vi "INIT swerve.vi"(8 "error in (no error)":errorcluster) -> (0 "error out":errorcluster)   [LabVIEW 2023]
uses:
  <vilib>/Rock Robotics/WPI/ThirdParty/REV Robotics/REVLib/Typedef/Spark MAX Control Type.ctl
  Global INIT.vi
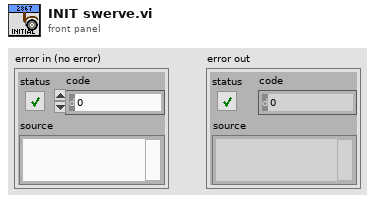
[diagram p1: front panel]
types:
  T1 = typedef "ctrl swerve motor.ctl" = cluster{"description":string, "MOTOR SELECT":T2, "Installed?":bool, "CAN ID":u8, "refnum name":string, "Invert":bool, "Idle Mode":T3, "Current limiting":T4, "MOTOR PIDF coefficients":T5, "gear ratio":dbl}
  T2 = typedef "ctrl MOTOR SELECT.ctl" = i16
  T3 = typedef "Spark MAX Idle Mode.ctl" = enum16{"Coast", "Brake"}
  T4 = typedef "ctrl Spark MAX current limiting.ctl" = cluster{"Linearized":bool, "Free Speed (A)":dbl, "Primay (A)":dbl, "Limit RPM (0)":u32}
  T5 = typedef "ctrl motor PIDF coefficients.ctl" = cluster{"PIDF":cluster{"P Gain":dbl, "I Gain":dbl, "D Gain":dbl, "F Gain":dbl, "I Zone":dbl, "Min Output":dbl, "Max Output":dbl}, "Smart Motion":T6}
  T6 = typedef "Spark MAX Smart Motion Parameters.ctl" = cluster{"Max Velocity":dbl, "Max Acceleration":dbl, "Minimum Velocity Output":dbl, "Allowed Closed Loop Error":dbl}
  T7 = typedef "ctrl CANcoder.ctl" = cluster{"description":string, "Installed?":bool, "CAN ID":u8, "CAN Bus":string, "refnum name":string, "Sensor Direction":bool, "Magnet Offset (Degrees)":dbl, "gear ratio":dbl}
  T8 = typedef "Spark MAX Control Type.ctl" = enum16{"Percent VBus", "Voltage", "Velocity", "Position", "Smart Motion", "Current", "Smart Velocity"}
  T9 = typedef "WPI_MotorControlDeviceRef.ctl" = cluster{"DeviceStatus":errorcluster, "Type":T10, "PWM":cluster{"PWM Channel":T11, "DeadBand":T12}, "CAN":cluster{"Device Number":u8, "SetOutput VI Ref":variant, "GetOutput VI Ref":variant, "Enable VI Ref":variant, "Disable VI Ref":variant, "Data":variant}, "Invert":bool, "DIO PWM":cluster{"PWM \"Enable\" Channel":T11, "DIOChannel":T13, "PWM Rate":dbl}}
  T10 = typedef "WPI_MotorControlType.ctl" = enum16{"PWM", "CAN", "DIO PWM"}
  T11 = typedef "FPGA_DIOPWMChannel.ctl" = enum8{"PWM 0", "PWM 1", "PWM 2", "PWM 3", "PWM 4", "PWM 5", "PWM 6", "PWM 7", "PWM 8", "PWM 9", "PWM MXP 0", "PWM MXP 1", "PWM MXP 2", "PWM MXP 3", "PWM MXP 4", "PWM MXP 5", "PWM MXP 6", "PWM MXP 7", "PWM MXP 8", "PWM MXP 9", "Invalid"}
  T12 = typedef "WPI_PWMDeadband.ctl" = cluster{"Name":string, "maxPositivePwm":i32, "minPositivePwm":i32, "centerPwm":i32, "maxNegativePwm":i32, "minNegativePwm":i32, "angularRange":u16}
  T13 = typedef "FPGA_DIOChannel.ctl" = enum8{"DIO 0", "DIO 1", "DIO 2", "DIO 3", "DIO 4", "DIO 5", "DIO 6", "DIO 7", "DIO 8", "DIO 9", "DIO MXP 0", "DIO MXP 1", "DIO MXP 2", "DIO MXP 3", "DIO MXP 4", "DIO MXP 5", "DIO MXP 6", "DIO MXP 7", "DIO MXP 8", "DIO MXP 9", "DIO MXP 10", "DIO MXP 11", "DIO MXP 12", "DIO MXP 13", "DIO MXP 14", "DIO MXP 15", "SPI Port CS1", "SPI Port CS2", "SPI Port CS3", "SPI Port MISO", "SPI Port MOSI", "Invalid"}
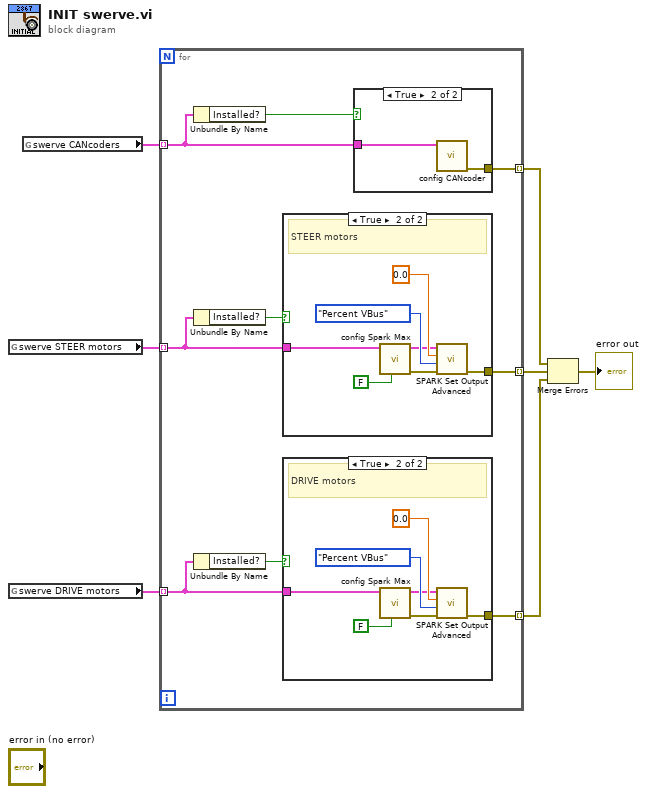
[diagram p0: block diagram]
diagram:
  n1 = global read "Global INIT.vi" "swerve STEER motors"() -> (w5:T1[])
  n2 = global read "Global INIT.vi" "swerve DRIVE motors"() -> (w7:T1[])
  n3 = global read "Global INIT.vi" "swerve CANcoders"() -> (w6:T7[])
  n4 = for {
    tunnel: w5 -> [w14] mode=indexing
    tunnel: w6 -> [w12] mode=indexing
    tunnel: w7 -> [w15] mode=indexing
    tunnel: [w10] -> w3 mode=indexing
    tunnel: [w9] -> w2 mode=indexing
    tunnel: [w8] -> w4 mode=indexing
    n5 = Unbundle By Name(w12) -> ("Installed?"=w11:bool)
    n6 = Unbundle By Name(w14) -> ("Installed?"=w13:bool)
    n7 = Unbundle By Name(w15) -> ("Installed?"=w16:bool)
    n8 = case shown="True" w13 {
      tunnel: w14 -> [_ w23]
      tunnel: [_ w19] -> w10
      frame False {
      }
      frame True {
        # "STEER motors"
        n9 = call "config Spark Max.vi"("LIMIT SW\nEnabled?"=FALSE ("LIMIT SW\nEnabled?"), "motor\ndefaults"=w23) -> ("error out"=w20:errorcluster, "MotorControlDevRef"=w21:T9)  [unwired: 8 in]
        n10 = call <vilib>:"SPARK Set Output Advanced.vi"("error in (no error)"=w20, "Control Mode"=Spark_MAX_Control_Type."Percent VBus", "Setpoint"=0.0 ("Output"), "MotorControlDevRef"=w21) -> ("error out"=w19:errorcluster)  [unwired: 6 in, 1 out]
      }
    }
    n11 = case shown="True" w16 {
      tunnel: w15 -> [_ w30]
      tunnel: [_ w26] -> w9
      frame False {
      }
      frame True {
        # "DRIVE motors"
        n12 = call "config Spark Max.vi"("LIMIT SW\nEnabled?"=FALSE ("LIMIT SW\nEnabled?"), "motor\ndefaults"=w30) -> ("error out"=w28:errorcluster, "MotorControlDevRef"=w29:T9)  [unwired: 8 in]
        n13 = call <vilib>:"SPARK Set Output Advanced.vi"("error in (no error)"=w28, "Control Mode"=Spark_MAX_Control_Type."Percent VBus", "Setpoint"=0.0 ("Output"), "MotorControlDevRef"=w29) -> ("error out"=w26:errorcluster)  [unwired: 6 in, 1 out]
      }
    }
    n14 = case shown="True" w11 {
      tunnel: w12 -> [_ w18]
      tunnel: [_ w17] -> w8
      frame False {
      }
      frame True {
        n15 = call "config CANcoder.vi"("CANcoder init data"=w18) -> ("error out"=w17:errorcluster)  [unwired: 10 in]
      }
    }
  }
  n16 = Merge Errors(w4, w3, w2) -> (→"error out":errorcluster)
